vi "Box_Scale.vi"(1 "Rectangle in":T1, 2 "Scale factor":dbl=1.0) -> (0 "Rectangle out":T1)   [LabVIEW 2018, in "Cage Diagram.lvlib"]
uses:
  Cage Diagram.lvlib
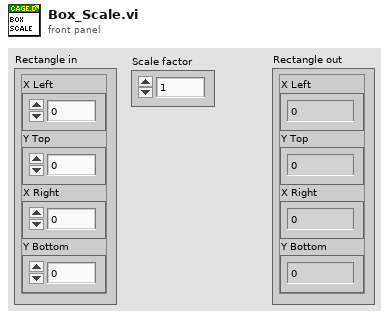
[diagram p1: front panel]
types:
  T1 = cluster{"X Left":i32, "Y Top":i32, "X Right":i32, "Y Bottom":i32}
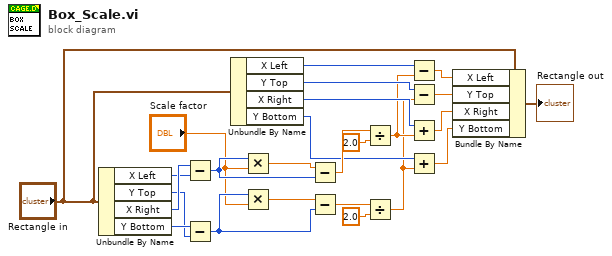
[diagram p0: block diagram]
diagram:
  n1 = Unbundle By Name("Rectangle in") -> ("X Left"=w24:i32, "Y Top"=w5:i32, "X Right"=w25:i32, "Y Bottom"=w6:i32)
  n2 = Subtract(x=w25, y=w24) -> (x-y=w22:i32)
  n3 = Subtract(x=w6, y=w5) -> (x-y=w4:i32)
  n4 = Unbundle By Name("Rectangle in") -> ("X Left"=w19:i32, "Y Top"=w18:i32, "X Right"=w17:i32, "Y Bottom"=w16:i32)
  n5 = Multiply(x=w22, y="Scale factor") -> (x*y=w23:dbl)
  n6 = Multiply(x=w4, y="Scale factor") -> (x*y=w7:dbl)
  n7 = Subtract(x=w23, y=w22) -> (x-y=w21:dbl)
  n8 = Subtract(x=w7, y=w4) -> (x-y=w8:dbl)
  n9 = Divide(x=w21, y=2.0) -> (x/y=w10:dbl)
  n10 = Divide(x=w8, y=2.0) -> (x/y=w2:dbl)
  n11 = Subtract(x=w19, y=w10) -> (x-y=w15:dbl)
  n12 = Subtract(x=w18, y=w2) -> (x-y=w14:dbl)
  n13 = Add(x=w17, y=w10) -> (x+y=w13:dbl)
  n14 = Add(x=w16, y=w2) -> (x+y=w12:dbl)
  n15 = Bundle By Name(cluster="Rectangle in", "X Left"=w15, "Y Top"=w14, "X Right"=w13, "Y Bottom"=w12) -> (→"Rectangle out":T1)
